vi "DSF.Engine.Execution.BuilderManager.Launch.vi"(8 "error in (no error)":errorcluster, 11 "Builder Manager in":refnum<class "DSF.Engine.Execution.BuilderManager.lvclass">) -> (0 "error out":errorcluster, 3 "Builder Manager out":refnum<class "DSF.Engine.Execution.BuilderManager.lvclass">)   [LabVIEW 2016, in "DSF.Engine.lvlib" / "DSF.Engine.Execution.BuilderManager.lvclass"]
uses:
  DSF.Engine.Execution.BuilderManager.lvclass
  DSF.Engine.Execution.BuilderManager.lvclass/DSF.Engine.Execution.BuilderManager.ctl
  Builder/DSF.Engine.Execution.Builder.lvclass
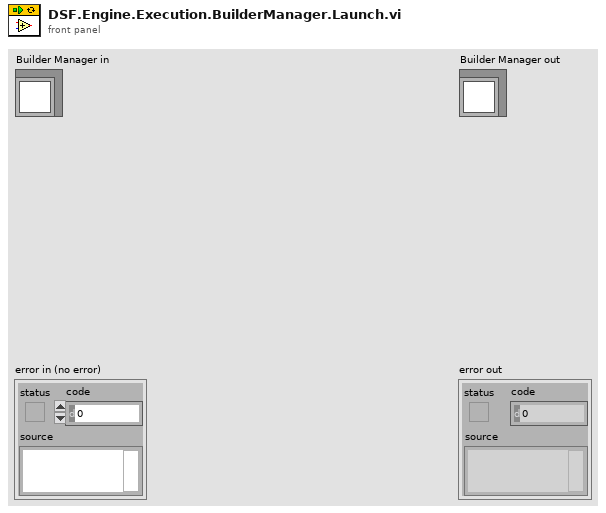
[diagram p1: front panel]
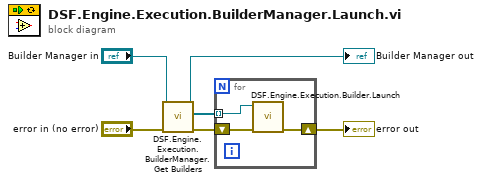
[diagram p0: block diagram]
diagram:
  n1 = call "DSF.Engine.Execution.BuilderManager.Get Builders.vi"("error in (no error)"="error in (no error)", "Builder Manager in"="Builder Manager in") -> ("error out"=w4:errorcluster, "Builders"=w2:refnum<class "DSF.Engine.Execution.Builder.lvclass">[], "Builder Manager out"=→"Builder Manager out":refnum<class "DSF.Engine.Execution.BuilderManager.lvclass">)  [unwired: 7 in]
  n2 = for {
    shift-right: [w8] -> w1
    shift-left: w4 -> [w9]
    tunnel: w2 -> [w7] mode=indexing
    n3 = call "DSF.Engine.Execution.Builder.Launch.vi"("error in (no error)"=w9, "Builder in"=w7) -> ("error out"=w8:errorcluster)  [unwired: 8 in, 1 out]
  }
  "error out" <- w1
